vi "Flywheels.vi"(0 "SP (RPM)":dbl=3000.0, 5 "P-gain":dbl=1e-05, 7 "Deadband (RPM)":dbl=10.0, 11 "error in (no error)":errorcluster) -> (3 "Flywheel Motors":dbl, 4 "PV (RPM)":dbl, 14 "Flywheels OK?":bool, 15 "error out":errorcluster)   [LabVIEW 2016]
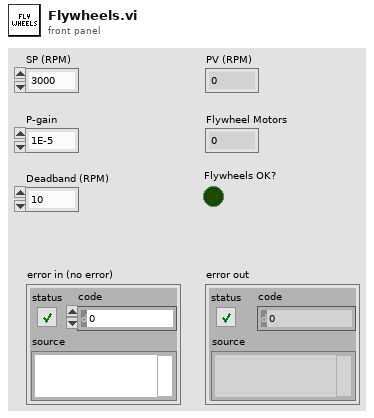
[diagram p1: front panel]
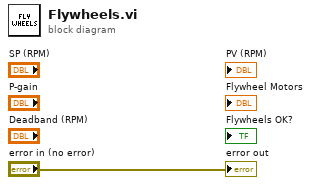
[diagram p0: block diagram]
diagram:
  "error out" <- "error in (no error)"
